vi "Get Modified.vi"(8 "error in (no error)":errorcluster caption="错误输入（无错误）", 11 "Generic输入":refnum<class "Generic.lvclass">) -> (0 "error out":errorcluster caption="错误输出", 2 "Modified":bool, 3 "Generic输出":refnum<class "Generic.lvclass">)   [LabVIEW 2013, in "Hierarchy Framework.lvlib" / "Generic.lvclass"]
uses:
  Generic.lvclass
  Generic.lvclass/Generic.ctl
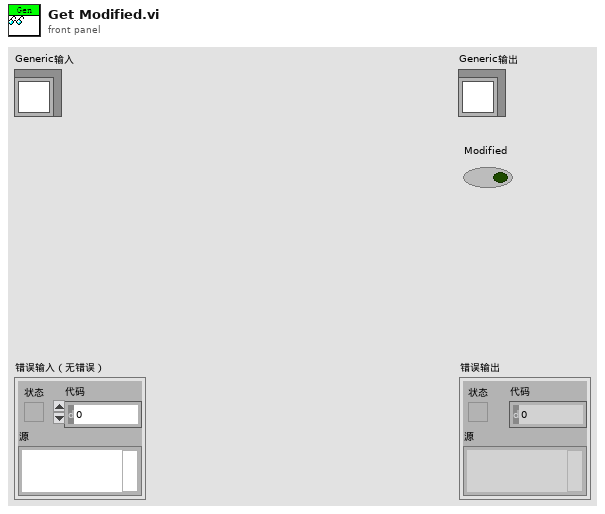
[diagram p1: front panel]
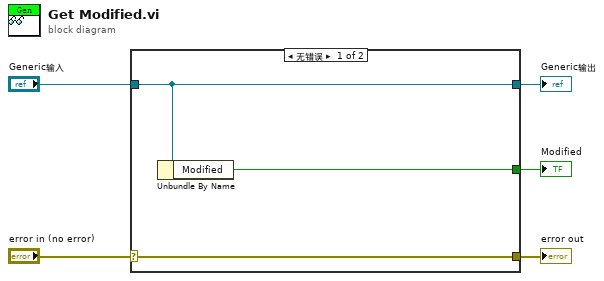
[diagram p0: block diagram]
diagram:
  n1 = case shown="无错误" "error in (no error)" {
    selector: "error in (no error)" -> [w8 w9]
    tunnel: [w8 w9] -> w4
    tunnel: [w7 w10] -> w2
    tunnel: "Generic输入" -> [w7 w10]
    tunnel: [w6 _] -> w1
    frame No Error {
      n2 = Unbundle By Name(w7) -> ("Modified"=w6:bool)
    }
    frame Error {
    }
  }
  "error out" <- w4
  "Generic输出" <- w2
  "Modified" <- w1
